vi "test TCX read (installed 71).vi"() -> ()   [LabVIEW 2011]
uses:
  XML Structure - Cluster.ctl
  XML Tag Type - Enum.ctl
panel:
  in  "Tree":string(tree)
  out "error out":errorcluster
  out "Attributes":cluster{"Keys":string[], "Values":string[]}
  out "child elements":i32[](array[numeric])
  in  "child name":string
  out "length":i32
  out "substring":string
  in  "tag index":i32
  out "xml structure":T1
  out "time":u32
  in  "text":string="<TrainingCenterDatabase xmlns=\"http://www.garmin.com/xmlschemas/TrainingCenterDatabase/v2\" xmlns:xsi=\"http://www.w3.org/2001/XMLSchema-instance\" xsi:schemaLocation=\"http://www.garmin.com/xmlschemas/TrainingCenterDatabase/v2 http://www.garmin.com/xmlschemas/TrainingCenterDatabasev2.xsd\"><Activities><Activity Sport=\"Biking\"><Id>2008-03-03T13:47:42Z</Id><Lap StartTime=\"2008-03-03T13:47:42Z\"><TotalTimeSeconds>1299.09</TotalTimeSeconds><DistanceMeters>11217.786133</DistanceMeters><MaximumSpeed>14.960000</MaximumSpeed><Calories>421</Calories><Intensity>Active</Intensity><Cadence>75</Cadence><TriggerMethod>Manual</TriggerMethod><Track><Trackpoint><Time>2008-03-03T13:47:42Z</Time><Position><LatitudeDegrees>35.889074</LatitudeDegrees><LongitudeDegrees>-78.952007</LongitudeDegrees></Position><AltitudeMeters>73.198</AltitudeMeters><DistanceMeters>0.000</DistanceMeters></Trackpoint><Trackpoint><Time>2008-03-03T13:47:43Z</Time><Position><LatitudeDegrees>35.889074</LatitudeDegrees><LongitudeDegrees>-78.952007</LongitudeDegrees></Position><AltitudeMeters>81.369</AltitudeMeters><DistanceMeters>0.006</DistanceMeters></Trackpoint><Trackpoint><Time>2008-03-03T13:47:44Z</Time><Position><LatitudeDegrees>35.889074</LatitudeDegrees><LongitudeDegrees>-78.952006</LongitudeDegrees></Position><AltitudeMeters>81.369</AltitudeMeters><DistanceMeters>0.032</DistanceMeters></Trackpoint><Trackpoint><Time>2008-03-03T13:47:45Z</Time><Position><LatitudeDegrees>35.889074</LatitudeDegrees><LongitudeDegrees>-78.952006</LongitudeDegrees></Position><AltitudeMeters>73.678</AltitudeMeters><DistanceMeters>0.039</DistanceMeters></Trackpoint><Trackpoint><Time>2008-03-03T13:47:46Z</Time><Position><LatitudeDegrees>35.889073</LatitudeDegrees><LongitudeDegrees>-78.952006</LongitudeDegrees></Position><AltitudeMeters>73.678</AltitudeMeters><DistanceMeters>0.039</DistanceMeters></Trackpoint><Trackpoint><Time>2008-03-03T13:47:47Z</Time><Position><LatitudeDegrees>35.889073</LatitudeDegrees><LongitudeDegrees>-78.952005</LongitudeDegrees></Position><AltitudeMeters>73.678</AltitudeMeters><DistanceMeters>0.039</DistanceMeters></Trackpoint><Trackpoint><Time>2008-03-03T13:47:48Z</Time><Position><LatitudeDegrees>35.889068</LatitudeDegrees><LongitudeDegrees>-78.951998</LongitudeDegrees></Position><AltitudeMeters>73.198</AltitudeMeters><DistanceMeters>0.979</DistanceMeters></Trackpoint><Trackpoint><Time>2008-03-03T13:47:49Z</Time><Position><LatitudeDegrees>35.889053</LatitudeDegrees><LongitudeDegrees>-78.951976</LongitudeDegrees></Position><AltitudeMeters>73.198</AltitudeMeters><DistanceMeters>3.587</DistanceMeters></Trackpoint><Trackpoint><Time>2008-03-03T13:47:50Z</Time><Position><LatitudeDegrees>35.889036</LatitudeDegrees><LongitudeDegrees>-78.951938</LongitudeDegrees></Position><AltitudeMeters>72.717</AltitudeMeters><DistanceMeters>7.581</DistanceMeters></Trackpoint><Trackpoint><Time>2008-03-03T13:47:51Z</Time><Position><LatitudeDegrees>35.889025</LatitudeDegrees><LongitudeDegrees>-78.951887</LongitudeDegrees></Position><AltitudeMeters>72.717</AltitudeMeters><DistanceMeters>12.400</DistanceMeters></Trackpoint><Trackpoint><Time>2008-03-03T13:47:52Z</Time><Position><LatitudeDegrees>35.889025</LatitudeDegrees><LongitudeDegrees>-78.951831</LongitudeDegrees></Position><AltitudeMeters>72.717</AltitudeMeters><DistanceMeters>17.352</DistanceMeters></Trackpoint><Trackpoint><Time>2008-03-03T13:47:53Z</Time><Position><LatitudeDegrees>35.889043</LatitudeDegrees><LongitudeDegrees>-78.951782</LongitudeDegrees></Position><AltitudeMeters>72.717</AltitudeMeters><DistanceMeters>22.277</DistanceMeters><Cadence>4</Cadence><Extensions><TPX xmlns=\"http://www.garmin.com/xmlschemas/ActivityExtension/v2\"><Watts>601</Watts></TPX></Extensions></Trackpoint><Trackpoint><Time>2008-03-03T13:47:54Z</Time><Position><LatitudeDegrees>35.889082</LatitudeDegrees><LongitudeDegrees>-78.951738</LongitudeDegrees></Position><AltitudeMeters>72.717</AltitudeMeters><DistanceMeters>28.108</DistanceMeters><Cadence>67</Cadence><Extensions><TPX xmlns=\"http://www.garmin.com/xmlschemas/ActivityExtension/v2\"><Watts>509</Watts></TPX></Extensions></Trackpoint><Trackpoint><Time>2008-03-03T13:47:55Z</Time><Position><LatitudeDegrees>35.889128</LatitudeDegrees><LongitudeDegrees>-78.951699</LongitudeDegrees></Position><AltitudeMeters>72.717</AltitudeMeters><DistanceMeters>34.434</DistanceMeters><Cadence>75</Cadence><Extensions><TPX xmlns=\"http://www.garmin.com/xmlschemas/ActivityExtension/v2\"><Watts>457</Watts></TPX></Extensions></Trackpoint><Trackpoint><Time>2008-03-03T13:47:56Z</Time><Position><LatitudeDegrees>35.889183</LatitudeDegrees><LongitudeDegrees>-78.951663</LongitudeDegrees></Position><AltitudeMeters>72.717</AltitudeMeters><DistanceMeters>41.291</DistanceMeters><Cadence>72</Cadence><Extensions><TPX xmlns=\"http://www.garmin.com/xmlschemas/ActivityExtension/v2\"><Watts>464</Watts></TPX></Extensions></Trackpoint><Trackpoint><Time>2008-03-03T13:47:57Z</Time><Position><LatitudeDegrees>35.889243</LatitudeDegrees><LongitudeDegrees>-78.951632</LongitudeDegrees></Position><AltitudeMeters>72.717</AltitudeMeters><DistanceMeters>48.540</DistanceMeters><Cadence>76</Cadence><Extensions><TPX xmlns=\"http://www.garmin.com/xmlschemas/ActivityExtension/v2\"><Watts>453</Watts></TPX></Extensions></Trackpoint><Trackpoint><Time>2008-03-03T13:47:58Z</Time><Position><LatitudeDegrees>35.889309</LatitudeDegrees><LongitudeDegrees>-78.951612</LongitudeDegrees></Position><AltitudeMeters>73.198</AltitudeMeters><DistanceMeters>56.120</DistanceMeters><Cadence>79</Cadence><Extensions><TPX xmlns=\"http://www.garmin.com/xmlschemas/ActivityExtension/v2\"><Watts>500</Watts></TPX></Extensions></Trackpoint><Trackpoint><Time>2008-03-03T13:47:59Z</Time><Position><LatitudeDegrees>35.889382</LatitudeDegrees><LongitudeDegrees>-78.951604</LongitudeDegrees></Position><AltitudeMeters>73.678</AltitudeMeters><DistanceMeters>64.164</DistanceMeters><Cadence>82</Cadence><Extensions><TPX xmlns=\"http://www.garmin.com/xmlschemas/ActivityExtension/v2\"><Watts>496</Watts></TPX></Extensions></Trackpoint><Trackpoint><Time>2008-03-03T13:48:00Z</Time><Position><LatitudeDegrees>35.889451</LatitudeDegrees><LongitudeDegrees>-78.951590</LongitudeDegrees></Position><AltitudeMeters>73.678</AltitudeMeters><DistanceMeters>71.959</DistanceMeters><Cadence>82</Cadence><Extensions><TPX xmlns=\"http://www.garmin.com/xmlschemas/ActivityExtension/v2\"><Watts>497</Watts></TPX></Extensions></Trackpoint><Trackpoint><Time>2008-03-03T13:48:01Z</Time><Position><LatitudeDegrees>35.889511</LatitudeDegrees><LongitudeDegrees>-78.951545</LongitudeDegrees></Position><AltitudeMeters>74.159</AltitudeMeters><DistanceMeters>79.567</DistanceMeters><Cadence>85</Cadence><Extensions><TPX xmlns=\"http://www.garmin.com/xmlschemas/ActivityExtension/v2\"><Watts>492</Watts></TPX></Extensions></Trackpoint><Trackpoint><Time>2008-03-03T13:48:02Z</Time><Position><LatitudeDegrees>35.889549</LatitudeDegrees><LongitudeDegrees>-78.951471</LongitudeDegrees></Position><AltitudeMeters>74.640</AltitudeMeters><DistanceMeters>87.343</DistanceMeters><Cadence>86</Cadence><Extensions><TPX xmlns=\"http://www.garmin.com/xmlschemas/ActivityExtension/v2\"><Watts>517</Watts></TPX></Extensions></Trackpoint><Trackpoint><Time>2008-03-03T13:48:03Z</Time><Position><LatitudeDegrees>35.889570</LatitudeDegrees><LongitudeDegrees>-78.951382</LongitudeDegrees></Position><AltitudeMeters>74.640</AltitudeMeters><DistanceMeters>95.795</DistanceMeters><Cadence>88</Cadence><Extensions><TPX xmlns=\"http://www.garmin.com/xmlschemas/ActivityExtension/v2\"><Watts>586</Watts></TPX></Extensions></Trackpoint><Trackpoint><Time>2008-03-03T13:48:04Z</Time><Position><LatitudeDegrees>35.889573</LatitudeDegrees><LongitudeDegrees>-78.951288</LongitudeDegrees></Position><AltitudeMeters>75.601</AltitudeMeters><DistanceMeters>104.176</DistanceMeters><Cadence>88</Cadence><Extensions><TPX xmlns=\"http://www.garmin.com/xmlschemas/ActivityExtension/v2\"><Watts>689</Watts></TPX></Extensions></Trackpoint><Trackpoint><Time>2008-03-03T13:48:05Z</Time><Position><LatitudeDegrees>35.889562</LatitudeDegrees><LongitudeDegrees>-78.951194</LongitudeDegrees></Position><AltitudeMeters>75.601</AltitudeMeters><DistanceMeters>112.762</DistanceMeters><Cadence>88</Cadence><Extensions><TPX xmlns=\"http://www.garmin.com/xmlschemas/ActivityExtension/v2\"><Watts>685</Watts></TPX></Extensions></Trackpoint><Trackpoint><Time>2008-03-03T13:48:06Z</Time><Position><LatitudeDegrees>35.889548</LatitudeDegrees><LongitudeDegrees>-78.951101</LongitudeDegrees></Position><AltitudeMeters>76.562</AltitudeMeters><DistanceMeters>121.305</DistanceMeters><Cadence>87</Cadence><Extensions><TPX xmlns=\"http://www.garmin.com/xmlschemas/ActivityExtension/v2\"><Watts>693</Watts></TPX></Extensions></Trackpoint><Trackpoint><Time>2008-03-03T13:48:07Z</Time><Position><LatitudeDegrees>35.889528</LatitudeDegrees><LongitudeDegrees>-78.951011</LongitudeDegrees></Position><AltitudeMeters>77.043</AltitudeMeters><DistanceMeters>129.784</DistanceMeters><Cadence>87</Cadence><Extensions><TPX xmlns=\"http://www.garmin.com/xmlschemas/ActivityExtension/v2\"><Watts>693</Watts></TPX></Extensions></Trackpoint><Trackpoint><Time>2008-03-03T13:48:08Z</Time><Position><LatitudeDegrees>35.889502</LatitudeDegrees><LongitudeDegrees>-78.950923</LongitudeDegrees></Position><AltitudeMeters>78.004</AltitudeMeters><DistanceMeters>138.261</DistanceMeters><Cadence>86</Cadence><Extensions><TPX xmlns=\"http://www.garmin.com/xmlschemas/ActivityExtension/v2\"><Watts>647</Watts></TPX></Extensions></Trackpoint><Trackpoint><Time>2008-03-03T13:48:09Z</Time><Position><LatitudeDegrees>35.889471</LatitudeDegrees><LongitudeDegrees>-78.950836</LongitudeDegrees></Position><AltitudeMeters>78.485</AltitudeMeters><DistanceMeters>146.753</DistanceMeters><Cadence>86</Cadence><Extensions><TPX xmlns=\"http://www.garmin.com/xmlschemas/ActivityExtension/v2\"><Watts>655</Watts></TPX></Extensions></Trackpoint><Trackpoint><Time>2008-03-03T13:48:10Z</Time><Position><LatitudeDegrees>35.889436</LatitudeDegrees><LongitudeDegrees>-78.950751</LongitudeDegrees></Position><AltitudeMeters>78.485</AltitudeMeters><DistanceMeters>155.350</DistanceMeters><Cadence>87</Cadence><Extensions><TPX xmlns=\"http://www.garmin.com/xmlschemas/ActivityExtension/v2\"><Watts>624</Watts></TPX></Extensions></Trackpoint><Trackpoint><Time>2008-03-03T13:48:11Z</Time><Position><LatitudeDegrees>35.889397</LatitudeDegrees><LongitudeDegrees>-78.950668</LongitudeDegrees></Position><AltitudeMeters>78.965</AltitudeMeters><DistanceMeters>164.034</DistanceMeters><Cadence>87</Cadence><Extensions><TPX xmlns=\"http://www.garmin.com/xmlschemas/ActivityExtension/v2\"><Watts>530</Watts></TPX></Extensions></Trackpoint><Trackpoint><Time>2008-03-03T13:48:12Z</Time><Position><LatitudeDegrees>35.889352</LatitudeDegrees><LongitudeDegrees>-78.950589</LongitudeDegrees></Position><AltitudeMeters>78.965</AltitudeMeters><DistanceMeters>172.768</DistanceMeters><Cadence>80</Cadence><Extensions><TPX xmlns=\"http://www.garmin.com/xmlschemas/ActivityExtension/v2\"><Watts>426</Watts></TPX></Extensions></Trackpoint><Trackpoint><Time>2008-03-03T13:48:13Z</Time><Position><LatitudeDegrees>35.889301</LatitudeDegrees><LongitudeDegrees>-78.950513</LongitudeDegrees></Position><AltitudeMeters>78.965</AltitudeMeters><DistanceMeters>181.637</DistanceMeters><Cadence>81</Cadence><Extensions><TPX xmlns=\"http://www.garmin.com/xmlschemas/ActivityExtension/v2\"><Watts>282</Watts></TPX></Extensions></Trackpoint><Trackpoint><Time>2008-03-03T13:48:14Z</Time><Position><LatitudeDegrees>35.889245</LatitudeDegrees><LongitudeDegrees>-78.950439</LongitudeDegrees></Position><AltitudeMeters>78.965</AltitudeMeters><DistanceMeters>190.815</DistanceMeters><Cadence>83</Cadence><Extensions><TPX xmlns=\"http://www.garmin.com/xmlschemas/ActivityExtension/v2\"><Watts>274</Watts></TPX></Extensions></Trackpoint><Trackpoint><Time>2008-03-03T13:48:15Z</Time><Position><LatitudeDegrees>35.889182</LatitudeDegrees><LongitudeDegrees>-78.950367</LongitudeDegrees></Position><AltitudeMeters>78.965</AltitudeMeters><DistanceMeters>200.345</DistanceMeters><Cadence>85</Cadence><Extensions><TPX xmlns=\"http://www.garmin.com/xmlschemas/ActivityExtension/v2\"><Watts>272</Watts></TPX></Extensions></Trackpoint><Trackpoint><Time>2008-03-03T13:48:16Z</Time><Position><LatitudeDegrees>35.889112</LatitudeDegrees><LongitudeDegrees>-78.950299</LongitudeDegrees></Position><AltitudeMeters>78.485</AltitudeMeters><DistanceMeters>210.272</DistanceMeters><Cadence>90</Cadence><Extensions><TPX xmlns=\"http://www.garmin.com/xmlschemas/ActivityExtension/v2\"><Watts>165</Watts></TPX></Extensions></Trackpoint><Trackpoint><Time>2008-03-03T13:48:17Z</Time><Position><LatitudeDegrees>35.889034</LatitudeDegrees><LongitudeDegrees>-78.950235</LongitudeDegrees></Position><AltitudeMeters>77.523</AltitudeMeters><DistanceMeters>220.744</DistanceMeters><Cadence>90</Cadence><Extensions><TPX xmlns=\"http://www.garmin.com/xmlschemas/ActivityExtension/v2\"><Watts>165</Watts></TPX></Extensions></Trackpoint><Trackpoint><Time>2008-03-03T13:48:18Z</Time><Position><LatitudeDegrees>35.888946</LatitudeDegrees><LongitudeDegrees>-78.950176</LongitudeDegrees></Position><AltitudeMeters>77.043</AltitudeMeters><DistanceMeters>231.911</DistanceMeters><Cadence>101</Cadence><Extensions><TPX xmlns=\"http://www.garmin.com/xmlschemas/ActivityExtension/v2\"><Watts>175</Watts></TPX></Extensions></Trackpoint><Trackpoint><Time>2008-03-03T13:48:19Z</Time><Position><LatitudeDegrees>35.888850</LatitudeDegrees><LongitudeDegrees>-78.950121</LongitudeDegrees></Position><AltitudeMeters>76.562</AltitudeMeters><DistanceMeters>243.635</DistanceMeters><Cadence>101</Cadence><Extensions><TPX xmlns=\"http://www.garmin.com/xmlschemas/ActivityExtension/v2\"><Watts>176</Watts></TPX></Extensions></Trackpoint><Trackpoint><Time>2008-03-03T13:48:20Z</Time><Position><LatitudeDegrees>35.888748</LatitudeDegrees><LongitudeDegrees>-78.950074</LongitudeDegrees></Position><AltitudeMeters>76.562</AltitudeMeters><DistanceMeters>255.800</DistanceMeters><Cadence>0</Cadence></Trackpoint><Trackpoint><Time>2008-03-03T13:48:21Z</Time><Position><LatitudeDegrees>35.888642</LatitudeDegrees><LongitudeDegrees>-78.950031</LongitudeDegrees></Position><AltitudeMeters>75.120</AltitudeMeters><DistanceMeters>268.157</DistanceMeters><Cadence>0</Cadence></Trackpoint><Trackpoint><Time>2008-03-03T13:48:22Z</Time><Position><LatitudeDegrees>35.888537</LatitudeDegrees><LongitudeDegrees>-78.949985</LongitudeDegrees></Position><AltitudeMeters>74.640</AltitudeMeters><DistanceMeters>280.559</DistanceMeters><Cadence>0</Cadence></Trackpoint><Trackpoint><Time>2008-03-03T13:48:23Z</Time><Position><LatitudeDegrees>35.888433</LatitudeDegrees><LongitudeDegrees>-78.949939</LongitudeDegrees></Position><AltitudeMeters>74.159</AltitudeMeters><DistanceMeters>292.870</DistanceMeters><Cadence>0</Cadence></Trackpoint><Trackpoint><Time>2008-03-03T13:48:24Z</Time><Position><LatitudeDegrees>35.888330</LatitudeDegrees><LongitudeDegrees>-78.949891</LongitudeDegrees></Position><AltitudeMeters>74.159</AltitudeMeters><DistanceMeters>305.059</DistanceMeters><Cadence>0</Cadence></Trackpoint><Trackpoint><Time>2008-03-03T13:48:25Z</Time><Position><LatitudeDegrees>35.888229</LatitudeDegrees><LongitudeDegrees>-78.949843</LongitudeDegrees></Position><AltitudeMeters>73.678</AltitudeMeters><DistanceMeters>317.013</DistanceMeters><Cadence>0</Cadence></Trackpoint><Trackpoint><Time>2008-03-03T13:48:26Z</Time><Position><LatitudeDegrees>35.888135</LatitudeDegrees><LongitudeDegrees>-78.949794</LongitudeDegrees></Position><AltitudeMeters>73.678</AltitudeMeters><DistanceMeters>328.272</DistanceMeters><Cadence>0</Cadence></Trackpoint><Trackpoint><Time>2008-03-03T13:48:27Z</Time><Position><LatitudeDegrees>35.888054</LatitudeDegrees><LongitudeDegrees>-78.949744</LongitudeDegrees></Position><AltitudeMeters>72.717</AltitudeMeters><DistanceMeters>338.319</DistanceMeters><Cadence>0</Cadence></Trackpoint><Trackpoint><Time>2008-03-03T13:48:28Z</Time><Position><LatitudeDegrees>35.887989</LatitudeDegrees><LongitudeDegrees>-78.949679</LongitudeDegrees></Position><AltitudeMeters>72.717</AltitudeMeters><DistanceMeters>347.512</DistanceMeters><Cadence>87</Cadence><Extensions><TPX xmlns=\"http://www.garmin.com/xmlschemas/ActivityExtension/v2\"><Watts>184</Watts></TPX></Extensions></Trackpoint><Trackpoint><Time>2008-03-03T13:48:29Z</Time><Position><LatitudeDegrees>35.887941</LatitudeDegrees><LongitudeDegrees>-78.949591</LongitudeDegrees></Position><AltitudeMeters>72.717</AltitudeMeters><DistanceMeters>357.049</DistanceMeters><Cadence>88</Cadence><Extensions><TPX xmlns=\"http://www.garmin.com/xmlschemas/ActivityExtension/v2\"><Watts>304</Watts></TPX></Extensions></Trackpoint><Trackpoint><Time>2008-03-03T13:48:30Z</Time><Position><LatitudeDegrees>35.887918</LatitudeDegrees><LongitudeDegrees>-78.949490</LongitudeDegrees></Position><AltitudeMeters>73.198</AltitudeMeters><DistanceMeters>366.543</DistanceMeters><Cadence>88</Cadence><Extensions><TPX xmlns=\"http://www.garmin.com/xmlschemas/ActivityExtension/v2\"><Watts>433</Watts></TPX></Extensions></Trackpoint><Trackpoint><Time>2008-03-03T13:48:31Z</Time><Position><LatitudeDegrees>35.887928</LatitudeDegrees><LongitudeDegrees>-78.949385</LongitudeDegrees></Position><AltitudeMeters>73.198</AltitudeMeters><DistanceMeters>376.010</DistanceMeters><Cadence>88</Cadence><Extensions><TPX xmlns=\"http://www.garmin.com/xmlschemas/ActivityExtension/v2\"><Watts>496</Watts></TPX></Extensions></Trackpoint><Trackpoint><Time>2008-03-03T13:48:32Z</Time><Position><LatitudeDegrees>35.887952</LatitudeDegrees><LongitudeDegrees>-78.949280</LongitudeDegrees></Position><AltitudeMeters>73.198</AltitudeMeters><DistanceMeters>385.936</DistanceMeters><Cadence>89</Cadence><Extensions><TPX xmlns=\"http://www.garmin.com/xmlschemas/ActivityExtension/v2\"><Watts>496</Watts></TPX></Extensions></Trackpoint><Trackpoint><Time>2008-03-03T13:48:33Z</Time><Position><LatitudeDegrees>35.887973</LatitudeDegrees><LongitudeDegrees>-78.949174</LongitudeDegrees></Position><AltitudeMeters>73.198</AltitudeMeters><DistanceMeters>395.759</DistanceMeters><Cadence>89</Cadence><Extensions><TPX xmlns=\"http://www.garmin.com/xmlschemas/ActivityExtension/v2\"><Watts>450</Watts></TPX></Extensions></Trackpoint><Trackpoint><Time>2008-03-03T13:48:34Z</Time><Position><LatitudeDegrees>35.887990</LatitudeDegrees><LongitudeDegrees>-78.949067</LongitudeDegrees></Position><AltitudeMeters>73.198</AltitudeMeters><DistanceMeters>405.530</DistanceMeters><Cadence>89</Cadence><Extensions><TPX xmlns=\"http://www.garmin.com/xmlschemas/ActivityExtension/v2\"><Watts>409</Watts></TPX></Extensions></Trackpoint><Trackpoint><Time>2008-03-03T13:48:35Z</Time><Position><LatitudeDegrees>35.888001</LatitudeDegrees><LongitudeDegrees>-78.948961</LongitudeDegrees></Position><AltitudeMeters>73.678</AltitudeMeters><DistanceMeters>415.221</DistanceMeters><Cadence>88</Cadence><Extensions><TPX xmlns=\"http://www.garmin.com/xmlschemas/ActivityExtension/v2\"><Watts>353</Watts></TPX></Extensions></Trackpoint><Trackpoint><Time>2008-03-03T13:48:36Z</Time><Position><LatitudeDegrees>35.888009</LatitudeDegrees><LongitudeDegrees>-78.948855</LongitudeDegrees></Position><AltitudeMeters>73.198</AltitudeMeters><DistanceMeters>424.794</DistanceMeters><Cadence>87</Cadence><Extensions><TPX xmlns=\"http://www.garmin.com/xmlschemas/ActivityExtension/v2\"><Watts>328</Watts></TPX></Extensions></Trackpoint><Trackpoint><Time>2008-03-03T13:48:37Z</Time><Position><LatitudeDegrees>35.888012</LatitudeDegrees><LongitudeDegrees>-78.948751</LongitudeDegrees></Position><AltitudeMeters>74.159</AltitudeMeters><DistanceMeters>434.220</DistanceMeters><Cadence>87</Cadence><Extensions><TPX xmlns=\"http://www.garmin.com/xmlschemas/ActivityExtension/v2\"><Watts>324</Watts></TPX></Extensions></Trackpoint><Trackpoint><Time>2008-03-03T13:48:38Z</Time><Position><LatitudeDegrees>35.888006</LatitudeDegrees><LongitudeDegrees>-78.948647</LongitudeDegrees></Position><AltitudeMeters>74.159</AltitudeMeters><DistanceMeters>443.557</DistanceMeters><Cadence>86</Cadence><Extensions><TPX xmlns=\"http://www.garmin.com/xmlschemas/ActivityExtension/v2\"><Watts>325</Watts></TPX></Extensions></Trackpoint><Trackpoint><Time>2008-03-03T13:48:39Z</Time><Position><LatitudeDegrees>35.887990</LatitudeDegrees><LongitudeDegrees>-78.948546</LongitudeDegrees></Position><AltitudeMeters>74.640</AltitudeMeters><DistanceMeters>452.875</DistanceMeters><Cadence>86</Cadence><Extensions><TPX xmlns=\"http://www.garmin.com/xmlschemas/ActivityExtension/v2\"><Watts>324</Watts></TPX></Extensions></Trackpoint><Trackpoint><Time>2008-03-03T13:48:40Z</Time><Position><LatitudeDegrees>35.887970</LatitudeDegrees><LongitudeDegrees>-78.948447</LongitudeDegrees></Position><AltitudeMeters>74.640</AltitudeMeters><DistanceMeters>462.057</DistanceMeters><Cadence>85</Cadence><Extensions><TPX xmlns=\"http://www.garmin.com/xmlschemas/ActivityExtension/v2\"><Watts>335</Watts></TPX></Extensions></Trackpoint><Trackpoint><Time>2008-03-03T13:48:41Z</Time><Position><LatitudeDegrees>35.887946</LatitudeDegrees><LongitudeDegrees>-78.948352</LongitudeDegrees></Position><AltitudeMeters>74.640</AltitudeMeters><DistanceMeters>471.034</DistanceMeters><Cadence>81</Cadence><Extensions><TPX xmlns=\"http://www.garmin.com/xmlschemas/ActivityExtension/v2\"><Watts>356</Watts></TPX></Extensions></Trackpoint><Trackpoint><Time>2008-03-03T13:48:42Z</Time><Position><LatitudeDegrees>35.887921</LatitudeDegrees><LongitudeDegrees>-78.948261</LongitudeDegrees></Position><AltitudeMeters>75.120</AltitudeMeters><DistanceMeters>479.710</DistanceMeters><Cadence>79</Cadence><Extensions><TPX xmlns=\"http://www.garmin.com/xmlschemas/ActivityExtension/v2\"><Watts>352</Watts></TPX></Extensions></Trackpoint><Trackpoint><Time>2008-03-03T13:48:43Z</Time><Position><LatitudeDegrees>35.887897</LatitudeDegrees><LongitudeDegrees>-78.948174</LongitudeDegrees></Position><AltitudeMeters>75.601</AltitudeMeters><DistanceMeters>488.013</DistanceMeters><Cadence>75</Cadence><Extensions><TPX xmlns=\"http://www.garmin.com/xmlschemas/ActivityExtension/v2\"><Watts>401</Watts></TPX></Extensions></Trackpoint><Trackpoint><Time>2008-03-03T13:48:44Z</Time><Position><LatitudeDegrees>35.887872</LatitudeDegrees><LongitudeDegrees>-78.948092</LongitudeDegrees></Position><AltitudeMeters>76.081</AltitudeMeters><DistanceMeters>495.870</DistanceMeters><Cadence>75</Cadence><Extensions><TPX xmlns=\"http://www.garmin.com/xmlschemas/ActivityExtension/v2\"><Watts>399</Watts></TPX></Extensions></Trackpoint><Trackpoint><Time>2008-03-03T13:48:45Z</Time><Position><LatitudeDegrees>35.887846</LatitudeDegrees><LongitudeDegrees>-78.948014</LongitudeDegrees></Position><AltitudeMeters>76.562</AltitudeMeters><DistanceMeters>503.435</DistanceMeters><Cadence>70</Cadence><Extensions><TPX xmlns=\"http://www.garmin.com/xmlschemas/ActivityExtension/v2\"><Watts>443</Watts></TPX></Extensions></Trackpoint><Trackpoint><Time>2008-03-03T13:48:46Z</Time><Position><LatitudeDegrees>35.887821</LatitudeDegrees><LongitudeDegrees>-78.947938</LongitudeDegrees></Position><AltitudeMeters>76.562</AltitudeMeters><DistanceMeters>510.811</DistanceMeters><Cadence>69</Cadence><Extensions><TPX xmlns=\"http://www.garmin.com/xmlschemas/ActivityExtension/v2\"><Watts>456</Watts></TPX></Extensions></Trackpoint><Trackpoint><Time>2008-03-03T13:48:47Z</Time><Position><LatitudeDegrees>35.887796</LatitudeDegrees><LongitudeDegrees>-78.947865</LongitudeDegrees></Position><AltitudeMeters>77.523</AltitudeMeters><DistanceMeters>517.950</DistanceMeters><Cadence>69</Cadence><Extensions><TPX xmlns=\"http://www.garmin.com/xmlschemas/ActivityExtension/v2\"><Watts>462</Watts></TPX></Extensions></Trackpoint><Trackpoint><Time>2008-03-03T13:48:48Z</Time><Position><LatitudeDegrees>35.887771</LatitudeDegrees><LongitudeDegrees>-78.947796</LongitudeDegrees></Position><AltitudeMeters>78.004</AltitudeMeters><DistanceMeters>524.769</DistanceMeters><Cadence>81</Cadence><Extensions><TPX xmlns=\"http://www.garmin.com/xmlschemas/ActivityExtension/v2\"><Watts>470</Watts></TPX></Extensions></Trackpoint><Trackpoint><Time>2008-03-03T13:48:49Z</Time><Position><LatitudeDegrees>35.887747</LatitudeDegrees><LongitudeDegrees>-78.947729</LongitudeDegrees></Position><AltitudeMeters>78.485</AltitudeMeters><DistanceMeters>531.361</DistanceMeters><Cadence>81</Cadence><Extensions><TPX xmlns=\"http://www.garmin.com/xmlschemas/ActivityExtension/v2\"><Watts>480</Watts></TPX></Extensions></Trackpoint><Trackpoint><Time>2008-03-03T13:48:50Z</Time><Position><LatitudeDegrees>35.887724</LatitudeDegrees><LongitudeDegrees>-78.947662</LongitudeDegrees></Position><AltitudeMeters>78.965</AltitudeMeters><DistanceMeters>537.959</DistanceMeters><Cadence>80</Cadence><Extensions><TPX xmlns=\"http://www.garmin.com/xmlschemas/ActivityExtension/v2\"><Watts>482</Watts></TPX></Extensions></Trackpoint><Trackpoint><Time>2008-03-03T13:48:51Z</Time><Position><LatitudeDegrees>35.887702</LatitudeDegrees><LongitudeDegrees>-78.947595</LongitudeDegrees></Position><AltitudeMeters>78.965</AltitudeMeters><DistanceMeters>544.500</DistanceMeters><Cadence>79</Cadence><Extensions><TPX xmlns=\"http://www.garmin.com/xmlschemas/ActivityExtension/v2\"><Watts>499</Watts></TPX></Extensions></Trackpoint><Trackpoint><Time>2008-03-03T13:48:52Z</Time><Position><LatitudeDegrees>35.887679</LatitudeDegrees><LongitudeDegrees>-78.947528</LongitudeDegrees></Position><AltitudeMeters>79.927</AltitudeMeters><DistanceMeters>551.001</DistanceMeters><Cadence>79</Cadence><Extensions><TPX xmlns=\"http://www.garmin.com/xmlschemas/ActivityExtension/v2\"><Watts>502</Watts></TPX></Extensions></Trackpoint><Trackpoint><Time>2008-03-03T13:48:53Z</Time><Position><LatitudeDegrees>35.887657</LatitudeDegrees><LongitudeDegrees>-78.947462</LongitudeDegrees></Position><AltitudeMeters>79.927</AltitudeMeters><DistanceMeters>557.480</DistanceMeters><Cadence>79</Cadence><Extensions><TPX xmlns=\"http://www.garmin.com/xmlschemas/ActivityExtension/v2\"><Watts>499</Watts></TPX></Extensions></Trackpoint><Trackpoint><Time>2008-03-03T13:48:54Z</Time><Position><LatitudeDegrees>35.887632</LatitudeDegrees><LongitudeDegrees>-78.947395</LongitudeDegrees></Position><AltitudeMeters>80.407</AltitudeMeters><DistanceMeters>564.096</DistanceMeters><Cadence>79</Cadence><Extensions><TPX xmlns=\"http://www.garmin.com/xmlschemas/ActivityExtension/v2\"><Watts>505</Watts></TPX></Extensions></Trackpoint><Trackpoint><Time>2008-03-03T13:48:55Z</Time><Position><LatitudeDegrees>35.887607</LatitudeDegrees><LongitudeDegrees>-78.947330</LongitudeDegrees></Position><AltitudeMeters>80.888</AltitudeMeters><DistanceMeters>570.617</DistanceMeters><Cadence>78</Cadence><Extensions><TPX xmlns=\"http://www.garmin.com/xmlschemas/ActivityExtension/v2\"><Watts>451</Watts></TPX></Extensions></Trackpoint><Trackpoint><Time>2008-03-03T13:48:56Z</Time><Position><LatitudeDegrees>35.887589</LatitudeDegrees><LongitudeDegrees>-78.947266</LongitudeDegrees></Position><AltitudeMeters>81.849</AltitudeMeters><DistanceMeters>576.695</DistanceMeters><Cadence>78</Cadence><Extensions><TPX xmlns=\"http://www.garmin.com/xmlschemas/ActivityExtension/v2\"><Watts>448</Watts></TPX></Extensions></Trackpoint><Trackpoint><Time>2008-03-03T13:48:57Z</Time><Position><LatitudeDegrees>35.887573</LatitudeDegrees><LongitudeDegrees>-78.947203</LongitudeDegrees></Position><AltitudeMeters>81.849</AltitudeMeters><DistanceMeters>582.599</DistanceMeters><Cadence>76</Cadence><Extensions><TPX xmlns=\"http://www.garmin.com/xmlschemas/ActivityExtension/v2\"><Watts>444</Watts></TPX></Extensions></Trackpoint><Trackpoint><Time>2008-03-03T13:48:58Z</Time><Position><LatitudeDegrees>35.887556</LatitudeDegrees><LongitudeDegrees>-78.947141</LongitudeDegrees></Position><AltitudeMeters>82.330</AltitudeMeters><DistanceMeters>588.498</DistanceMeters><Cadence>73</Cadence><Extensions><TPX xmlns=\"http://www.garmin.com/xmlschemas/ActivityExtension/v2\"><Watts>425</Watts></TPX></Extensions></Trackpoint><Trackpoint><Time>2008-03-03T13:48:59Z</Time><Position><LatitudeDegrees>35.887537</LatitudeDegrees><LongitudeDegrees>-78.947080</LongitudeDegrees></Position><AltitudeMeters>82.811</AltitudeMeters><DistanceMeters>594.422</DistanceMeters><Cadence>73</Cadence><Extensions><TPX xmlns=\"http://www.garmin.com/xmlschemas/ActivityExtension/v2\"><Watts>429</Watts></TPX></Extensions></Trackpoint><Trackpoint><Time>2008-03-03T13:49:00Z</Time><Position><LatitudeDegrees>35.887517</LatitudeDegrees><LongitudeDegrees>-78.947019</LongitudeDegrees></Position><AltitudeMeters>83.291</AltitudeMeters><DistanceMeters>600.405</DistanceMeters><Cadence>72</Cadence><Extensions><TPX xmlns=\"http://www.garmin.com/xmlschemas/ActivityExtension/v2\"><Watts>411</Watts></TPX></Extensions></Trackpoint><Trackpoint><Time>2008-03-03T13:49:01Z</Time><Position><LatitudeDegrees>35.887497</LatitudeDegrees><LongitudeDegrees>-78.946957</LongitudeDegrees></Position><AltitudeMeters>83.291</AltitudeMeters><DistanceMeters>606.405</DistanceMeters><Cadence>72</Cadence><Extensions><TPX xmlns=\"http://www.garmin.com/xmlschemas/ActivityExtension/v2\"><Watts>389</Watts></TPX></Extensions></Trackpoint><Trackpoint><Time>2008-03-03T13:49:02Z</Time><Position><LatitudeDegrees>35.887476</LatitudeDegrees><LongitudeDegrees>-78.946895</LongitudeDegrees></Position><AltitudeMeters>83.772</AltitudeMeters><DistanceMeters>612.437</DistanceMeters><Cadence>72</Cadence><Extensions><TPX xmlns=\"http://www.garmin.com/xmlschemas/ActivityExtension/v2\"><Watts>373</Watts></TPX></Extensions></Trackpoint><Trackpoint><Time>2008-03-03T13:49:03Z</Time><Position><LatitudeDegrees>35.887455</LatitudeDegrees><LongitudeDegrees>-78.946834</LongitudeDegrees></Position><AltitudeMeters>84.253</AltitudeMeters><DistanceMeters>618.473</DistanceMeters><Cadence>72</Cadence><Extensions><TPX xmlns=\"http://www.garmin.com/xmlschemas/ActivityExtension/v2\"><Watts>301</Watts></TPX></Extensions></Trackpoint><Trackpoint><Time>2008-03-03T13:49:04Z</Time><Position><LatitudeDegrees>35.887432</LatitudeDegrees><LongitudeDegrees>-78.946773</LongitudeDegrees></Position><AltitudeMeters>84.253</AltitudeMeters><DistanceMeters>624.463</DistanceMeters><Cadence>72</Cadence><Extensions><TPX xmlns=\"http://www.garmin.com/xmlschemas/ActivityExtension/v2\"><Watts>305</Watts></TPX></Extensions></Trackpoint><Trackpoint><Time>2008-03-03T13:49:05Z</Time><Position><LatitudeDegrees>35.887410</LatitudeDegrees><LongitudeDegrees>-78.946712</LongitudeDegrees></Position><AltitudeMeters>84.253</AltitudeMeters><DistanceMeters>630.534</DistanceMeters><Cadence>73</Cadence><Extensions><TPX xmlns=\"http://www.garmin.com/xmlschemas/ActivityExtension/v2\"><Watts>219</Watts></TPX></Extensions></Trackpoint><Trackpoint><Time>2008-03-03T13:49:06Z</Time><Position><LatitudeDegrees>35.887386</LatitudeDegrees><LongitudeDegrees>-78.946652</LongitudeDegrees></Position><AltitudeMeters>84.253</AltitudeMeters><DistanceMeters>636.573</DistanceMeters><Cadence>72</Cadence><Extensions><TPX xmlns=\"http://www.garmin.com/xmlschemas/ActivityExtension/v2\"><Watts>198</Watts></TPX></Extensions></Trackpoint><Trackpoint><Time>2008-03-03T13:49:07Z</Time><Position><LatitudeDegrees>35.887357</LatitudeDegrees><LongitudeDegrees>-78.946595</LongitudeDegrees></Position><AltitudeMeters>84.733</AltitudeMeters><DistanceMeters>642.613</DistanceMeters><Cadence>73</Cadence><Extensions><TPX xmlns=\"http://www.garmin.com/xmlschemas/ActivityExtension/v2\"><Watts>191</Watts></TPX></Extensions></Trackpoint><Trackpoint><Time>2008-03-03T13:49:08Z</Time><Position><LatitudeDegrees>35.887322</LatitudeDegrees><LongitudeDegrees>-78.946544</LongitudeDegrees></Position><AltitudeMeters>84.733</AltitudeMeters><DistanceMeters>648.631</DistanceMeters><Cadence>72</Cadence><Extensions><TPX xmlns=\"http://www.garmin.com/xmlschemas/ActivityExtension/v2\"><Watts>176</Watts></TPX></Extensions></Trackpoint><Trackpoint><Time>2008-03-03T13:49:09Z</Time><Position><LatitudeDegrees>35.887283</LatitudeDegrees><LongitudeDegrees>-78.946497</LongitudeDegrees></Position><AltitudeMeters>84.733</AltitudeMeters><DistanceMeters>654.684</DistanceMeters><Cadence>72</Cadence><Extensions><TPX xmlns=\"http://www.garmin.com/xmlschemas/ActivityExtension/v2\"><Watts>167</Watts></TPX></Extensions></Trackpoint><Trackpoint><Time>2008-03-03T13:49:10Z</Time><Position><LatitudeDegrees>35.887245</LatitudeDegrees><LongitudeDegrees>-78.946449</LongitudeDegrees></Position><AltitudeMeters>85.214</AltitudeMeters><DistanceMeters>660.752</DistanceMeters><Cadence>72</Cadence><Extensions><TPX xmlns=\"http://www.garmin.com/xmlschemas/ActivityExtension/v2\"><Watts>148</Watts></TPX></Extensions></Trackpoint><Trackpoint><Time>2008-03-03T13:49:11Z</Time><Position><LatitudeDegrees>35.887217</LatitudeDegrees><LongitudeDegrees>-78.946392</LongitudeDegrees></Position><AltitudeMeters>85.214</AltitudeMeters><DistanceMeters>666.765</DistanceMeters><Cadence>73</Cadence><Extensions><TPX xmlns=\"http://www.garmin.com/xmlschemas/ActivityExtension/v2\"><Watts>132</Watts></TPX></Extensions></Trackpoint><Trackpoint><Time>2008-03-03T13:49:12Z</Time><Position><LatitudeDegrees>35.887205</LatitudeDegrees><LongitudeDegrees>-78.946325</LongitudeDegrees></Position><AltitudeMeters>85.214</AltitudeMeters><DistanceMeters>672.852</DistanceMeters><Cadence>75</Cadence><Extensions><TPX xmlns=\"http://www.garmin.com/xmlschemas/ActivityExtension/v2\"><Watts>111</Watts></TPX></Extensions></Trackpoint><Trackpoint><Time>2008-03-03T13:49:13Z</Time><Position><LatitudeDegrees>35.887220</LatitudeDegrees><LongitudeDegrees>-78.946261</LongitudeDegrees></Position><AltitudeMeters>85.214</AltitudeMeters><DistanceMeters>678.848</DistanceMeters><Cadence>76</Cadence><Extensions><TPX xmlns=\"http://www.garmin.com/xmlschemas/ActivityExtension/v2\"><Watts>151</Watts></TPX></Extensions></Trackpoint><Trackpoint><Time>2008-03-03T13:49:14Z</Time><Position><LatitudeDegrees>35.887246</LatitudeDegrees><LongitudeDegrees>-78.946203</LongitudeDegrees></Position><AltitudeMeters>85.695</AltitudeMeters><DistanceMeters>684.743</DistanceMeters><Cadence>76</Cadence><Extensions><TPX xmlns=\"http://www.garmin.com/xmlschemas/ActivityExtension/v2\"><Watts>152</Watts></TPX></Extensions></Trackpoint><Trackpoint><Time>2008-03-03T13:49:15Z</Time><Position><LatitudeDegrees>35.887279</LatitudeDegrees><LongitudeDegrees>-78.946150</LongitudeDegrees></Position><AltitudeMeters>85.695</AltitudeMeters><DistanceMeters>690.774</DistanceMeters><Cadence>72</Cadence><Extensions><TPX xmlns=\"http://www.garmin.com/xmlschemas/ActivityExtension/v2\"><Watts>189</Watts></TPX></Extensions></Trackpoint><Trackpoint><Time>2008-03-03T13:49:16Z</Time><Position><LatitudeDegrees>35.887305</LatitudeDegrees><LongitudeDegrees>-78.946092</LongitudeDegrees></Position><AltitudeMeters>85.695</AltitudeMeters><DistanceMeters>696.757</DistanceMeters><Cadence>73</Cadence><Extensions><TPX xmlns=\"http://www.garmin.com/xmlschemas/ActivityExtension/v2\"><Watts>188</Watts></TPX></Extensions></Trackpoint><Trackpoint><Time>2008-03-03T13:49:17Z</Time><Position><LatitudeDegrees>35.887324</LatitudeDegrees><LongitudeDegrees>-78.946030</LongitudeDegrees></Position><AltitudeMeters>85.695</AltitudeMeters><DistanceMeters>702.740</DistanceMeters><Cadence>71</Cadence><Extensions><TPX xmlns=\"http://www.garmin.com/xmlschemas/ActivityExtension/v2\"><Watts>189</Watts></TPX></Extensions></Trackpoint><Trackpoint><Time>2008-03-03T13:49:18Z</Time><Position><LatitudeDegrees>35.887337</LatitudeDegrees><LongitudeDegrees>-78.945965</LongitudeDegrees></Position><AltitudeMeters>86.175</AltitudeMeters><DistanceMeters>708.772</DistanceMeters><Cadence>71</Cadence><Extensions><TPX xmlns=\"http://www.garmin.com/xmlschemas/ActivityExtension/v2\"><Watts>187</Watts></TPX></Extensions></Trackpoint><Trackpoint><Time>2008-03-03T13:49:19Z</Time><Position><LatitudeDegrees>35.887348</LatitudeDegrees><LongitudeDegrees>-78.945900</LongitudeDegrees></Position><AltitudeMeters>86.175</AltitudeMeters><DistanceMeters>714.821</DistanceMeters><Cadence>71</Cadence><Extensions><TPX xmlns=\"http://www.garmin.com/xmlschemas/ActivityExtension/v2\"><Watts>184</Watts></TPX></Extensions></Trackpoint><Trackpoint><Time>2008-03-03T13:49:20Z</Time><Position><LatitudeDegrees>35.887358</LatitudeDegrees><LongitudeDegrees>-78.945832</LongitudeDegrees></Position><AltitudeMeters>86.175</AltitudeMeters><DistanceMeters>721.001</DistanceMeters><Cadence>73</Cadence><Extensions><TPX xmlns=\"http://www.garmin.com/xmlschemas/ActivityExtension/v2\"><Watts>185</Watts></TPX></Extensions></Trackpoint><Trackpoint><Time>2008-03-03T13:49:21Z</Time><Position><LatitudeDegrees>35.887366</LatitudeDegrees><LongitudeDegrees>-78.945763</LongitudeDegrees></Position><AltitudeMeters>86.175</AltitudeMeters><DistanceMeters>727.328</DistanceMeters><Cadence>73</Cadence><Extensions><TPX xmlns=\"http://www.garmin.com/xmlschemas/ActivityExtension/v2\"><Watts>184</Watts></TPX></Extensions></Trackpoint><Trackpoint><Time>2008-03-03T13:49:22Z</Time><Position><LatitudeDegrees>35.887374</LatitudeDegrees><LongitudeDegrees>-78.945692</LongitudeDegrees></Position><AltitudeMeters>86.175</AltitudeMeters><DistanceMeters>733.782</DistanceMeters><Cadence>77</Cadence><Extensions><TPX xmlns=\"http://www.garmin.com/xmlschemas/ActivityExtension/v2\"><Watts>158</Watts></TPX></Extensions></Trackpoint><Trackpoint><Time>2008-03-03T13:49:23Z</Time><Position><LatitudeDegrees>35.887380</LatitudeDegrees><LongitudeDegrees>-78.945620</LongitudeDegrees></Position><AltitudeMeters>86.175</AltitudeMeters><DistanceMeters>740.379</DistanceMeters><Cadence>70</Cadence><Extensions><TPX xmlns=\"http://www.garmin.com/xmlschemas/ActivityExtension/v2\"><Watts>130</Watts></TPX></Extensions></Trackpoint><Trackpoint><Time>2008-03-03T13:49:24Z</Time><Position><LatitudeDegrees>35.887386</LatitudeDegrees><LongitudeDegrees>-78.945545</LongitudeDegrees></Position><AltitudeMeters>86.175</AltitudeMeters><DistanceMeters>747.240</DistanceMeters><Cadence>70</Cadence><Extensions><TPX xmlns=\"http://www.garmin.com/xmlschemas/ActivityExtension/v2\"><Watts>130</Watts></TPX></Extensions></Trackpoint><Trackpoint><Time>2008-03-03T13:49:25Z</Time><Position><LatitudeDegrees>35.887390</LatitudeDegrees><LongitudeDegrees>-78.945466</LongitudeDegrees></Position><AltitudeMeters>86.175</AltitudeMeters><DistanceMeters>754.348</DistanceMeters><Cadence>73</Cadence><Extensions><TPX xmlns=\"http://www.garmin.com/xmlschemas/ActivityExtension/v2\"><Watts>160</Watts></TPX></Extensions></Trackpoint><Trackpoint><Time>2008-03-03T13:49:26Z</Time><Position><LatitudeDegrees>35.887393</LatitudeDegrees><LongitudeDegrees>-78.945383</LongitudeDegrees></Position><AltitudeMeters>86.175</AltitudeMeters><DistanceMeters>761.841</DistanceMeters><Cadence>76</Cadence><Extensions><TPX xmlns=\"http://www.garmin.com/xmlschemas/ActivityExtension/v2\"><Watts>178</Watts></TPX></Extensions></Trackpoint><Trackpoint><Time>2008-03-03T13:49:27Z</Time><Position><LatitudeDegrees>35.887393</LatitudeDegrees><LongitudeDegrees>-78.945298</LongitudeDegrees></Position><AltitudeMeters>85.695</AltitudeMeters><DistanceMeters>769.610</DistanceMeters><Cadence>80</Cadence><Extensions><TPX xmlns=\"http://www.garmin.com/xmlschemas/ActivityExtension/v2\"><Watts>158</Watts></TPX></Extensions></Trackpoint><Trackpoint><Time>2008-03-03T13:49:28Z</Time><Position><LatitudeDegrees>35.887391</LatitudeDegrees><LongitudeDegrees>-78.945209</LongitudeDegrees></Position><AltitudeMeters>85.695</AltitudeMeters><DistanceMeters>777.621</DistanceMeters><Cadence>82</Cadence><Extensions><TPX xmlns=\"http://www.garmin.com/xmlschemas/ActivityExtension/v2\"><Watts>138</Watts></TPX></Extensions></Trackpoint><Trackpoint><Time>2008-03-03T13:49:29Z</Time><Position><LatitudeDegrees>35.887389</LatitudeDegrees><LongitudeDegrees>-78.945120</LongitudeDegrees></Position><AltitudeMeters>85.695</AltitudeMeters><DistanceMeters>785.702</DistanceMeters><Cadence>83</Cadence><Extensions><TPX xmlns=\"http://www.garmin.com/xmlschemas/ActivityExten
